vi "Untitled 22.vi"() -> ()   [LabVIEW 2019]
uses:
  Generated_client/RPC Messages/routeguide_Point.ctl
  Generated_client/RPC Messages/routeguide_Feature.ctl
  Generated_client/Generated_client.lvlib
panel:
  out "error out":errorcluster
  out "Response Data":T1
  in  "Request Data":T2
  in  "address":string
  in  "error in":errorcluster
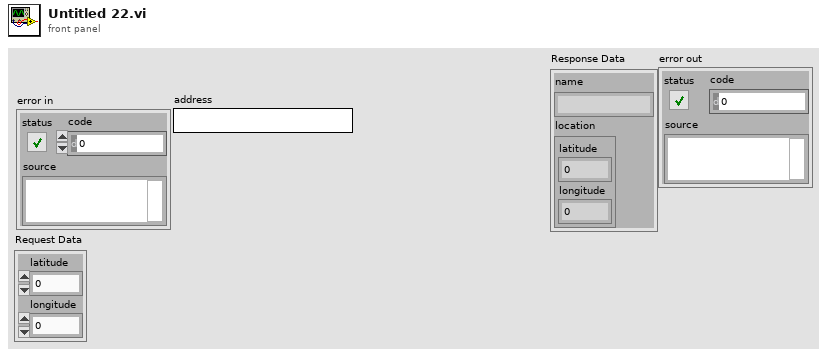
[diagram p1: front panel]
types:
  T1 = typedef "Generated_client.lvlib/routeguide_Feature.ctl" = cluster{"name":string, "location":T2}
  T2 = typedef "Generated_client.lvlib/routeguide_Point.ctl" = cluster{"latitude":i32, "longitude":i32}
  T3 = typedef "grpc-lvsupport-release.lvlib/grpcId.ctl" = u64
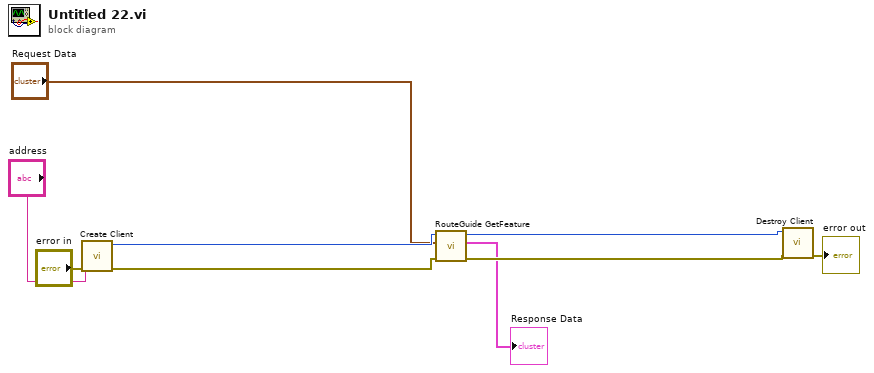
[diagram p0: block diagram]
diagram:
  n1 = call "Create Client.vi"("error in"="error in", "address"="address") -> ("error out"=w7:errorcluster, "gRPC ID Out"=w9:T3)  [unwired: 8 in]
  n2 = call "RouteGuide GetFeature.vi"("error in"=w7, "Request Data"="Request Data", "gRPC ID"=w9) -> ("error out"=w6:errorcluster, "Response Data"=→"Response Data":T1, "gRPC ID out"=w8:T3)  [unwired: 6 in]
  n3 = call "Destroy Client.vi"("error in"=w6, "gRPC ID"=w8) -> ("error out"=→"error out":errorcluster)  [unwired: 9 in]
